vi "Global settings termica.vi"() -> ()   [LabVIEW 2019]
uses:
  Cluster termica.ctl
panel:
  in  "Cluster termica":T1={"Tipo di servizio"=0, "s1"={"Intervallo fermate"=0.0}, "s3"={"Tempo a carico"=1.0, "Tempo a riposo"=1.0}, "Tempo prova max"=5.0, "Tempo acq auto"=1.0, "Escludi mis res se stop"=FALSE} {"Tempo acq auto" min=0.5 max=45.0 format="%#_g min"; "Tempo prova max" min=1.0 max=250.0 format="%#_g min"; "s3"."Tempo a riposo" min=1.0 format="%#_g min"; "s3"."Tempo a carico" min=1.0 format="%#_g min"; "s1"."Intervallo fermate" format="%#_g min"; "Tipo di servizio" items=["S1", "S3"]}
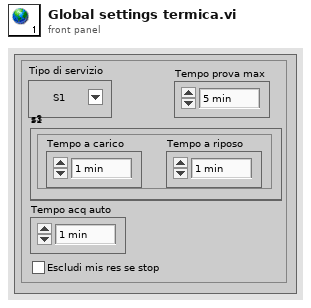
[diagram p1: front panel]
types:
  T1 = typedef "Cluster termica.ctl" = cluster{"Tipo di servizio":u16, "s1":cluster{"Intervallo fermate":dbl}, "s3":cluster{"Tempo a carico":dbl, "Tempo a riposo":dbl}, "Tempo prova max":dbl, "Tempo acq auto":dbl, "Escludi mis res se stop":bool}
diagram:
